vi "PROTECAO_DEC_UTILS.vi"(11 "Destino DEC":dbl) -> (3 "CONT DEC":i32)   [LabVIEW 2018]
uses:
  Global_Telescopio.vi
panel:
  out "DIST DEC":dbl
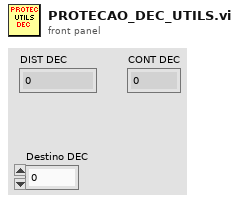
[diagram p1: front panel]
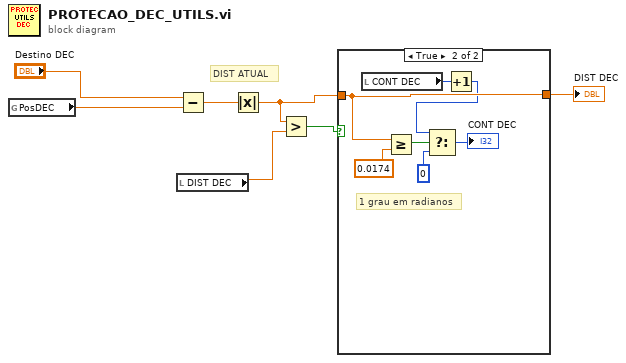
[diagram p0: block diagram]
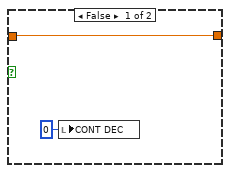
[diagram p2: hidden frame]
diagram:
  # "DIST ATUAL"
  n1 = global read "Global_Telescopio.vi" "PosDEC"() -> (w7:dbl)
  n2 = local read "DIST DEC"() -> (w3:dbl)
  n3 = Subtract(x="Destino DEC", y=w7) -> (x-y=w6:dbl)
  n4 = Absolute Value(x=w6) -> (abs(x)=w2:dbl)
  n5 = Greater?(x=w2, y=w3) -> (0:w4:bool)
  n6 = case shown="True" w4 {
    tunnel: w2 -> [w9 w16]
    tunnel: [w9 w16] -> w5
    frame False {
      n7 = local write "CONT DEC"(0 ("CONT AH")) -> ()
    }
    frame True {
      # "1 grau em radianos"
      n8 = local read "CONT DEC"() -> (w11:i32)
      n9 = Greater Or Equal?(x=w16, y=0.0174) -> (x >= y?=w14:bool)
      n10 = Increment(x=w11) -> (x+1=w10:i32)
      n11 = Select(t=w10, s=w14, f=0 ("t")) -> (s? t:f=→"CONT DEC":i32)
    }
  }
  "DIST DEC" <- w5
